vi "NumPad-ByRef.vi"(5 "Config":T1={"Title"="", "Minimum"=nan, "Maximum"=nan, "Decimals"=-1} {"Decimals" min=-1 max=6}, 6 "error in (no error)":errorcluster, 8 "device ID":refnum<k1>, 9 "NumericRef":refnum<vi>) -> (0 "error out":errorcluster, 2 "SetValue":dbl format="%#_8f", 3 "NumericRef out":refnum<vi>)   [LabVIEW 2016]
doc: "This subVI opens a number pad dialog to update the value to the referenced control.\nConfig cluster sets the title, max, min and number of decimal places. If config is not connected or any value is undefined, then the caption, max, min and increment of the referenced control are used.\n\nNOTE: The referenced control MUST have a caption set for LV8.5 !!!\n\n2-JAN-2008 R.Gibson"
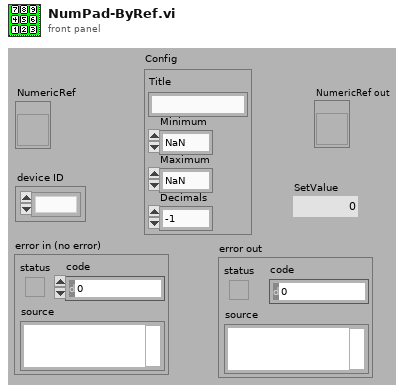
[diagram p1: front panel]
types:
  T1 = cluster{"Title":string, "Minimum":dbl, "Maximum":dbl, "Decimals":i8}
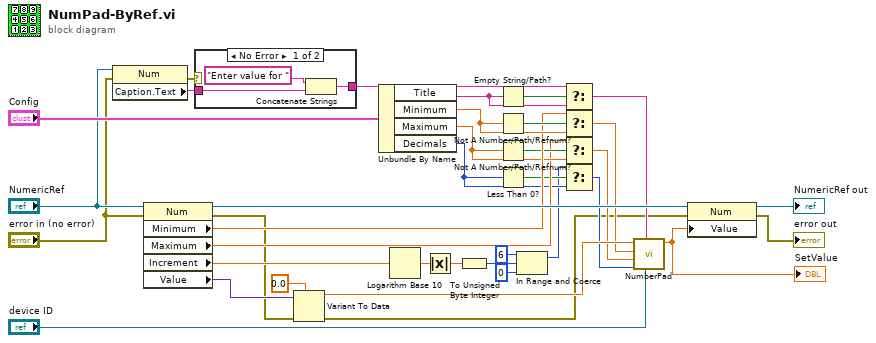
[diagram p0: block diagram]
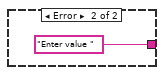
[diagram p2: hidden frame]
diagram:
  n1 = property on="Property Node" class="Num"(reference="NumericRef", error in="error in (no error)") -> (error out=w7:errorcluster, "Caption.Text"=w5:string)  [unwired: 1 out]
  n2 = property on="Property Node" class="Num"(reference="NumericRef", error in="error in (no error)") -> (reference out=w34:refnum<vi>, error out=w2:errorcluster, "Minimum"=w23:dbl, "Maximum"=w19:dbl, "Increment"=w35:dbl, "Value"=w6:variant)
  n3 = case shown="No Error" w7 {
    tunnel: w5 -> [w39 _]
    tunnel: [w38 "Enter value " ("Caption.Text")] -> w4
    frame No Error {
      n4 = Concatenate Strings("Enter value for " ("string"), w39) -> (w38:string)
    }
    frame Error {
    }
  }
  n5 = Variant To Data(error in=w2, type=0.0, Variant=w6) -> (data=w32:dbl, error out=w1:errorcluster)
  n6 = Unbundle By Name("Config") -> ("Title"=w27:string, "Minimum"=w24:dbl, "Maximum"=w20:dbl, "Decimals"=w16:i8)
  n7 = Logarithm Base 10(1:w35) -> (0:w36:dbl)
  n8 = Absolute Value(x=w36) -> (abs(x)=w14:dbl)
  n9 = To Unsigned Byte Integer(number=w14) -> (unsigned 8bit integer=w10:u8)
  n10 = Empty String/Path?(string/path=w27) -> (empty?=w28:bool)
  n11 = Not A Number/Path/Refnum?(number/path/refnum=w24) -> (NaN/Path/Refnum?=w25:bool)
  n12 = Not A Number/Path/Refnum?(number/path/refnum=w20) -> (NaN/Path/Refnum?=w21:bool)
  n13 = Less Than 0?(x=w16) -> (x < 0?=w15:bool)
  n14 = In Range and Coerce(upper limit=u8 6, x=w10, lower limit=u8 0) -> (coerced(x)=w13:u8)  [unwired: 1 out]
  n15 = Select(t=w4, s=w28, f=w27) -> (s? t:f=w26:string)
  n16 = Select(t=w23, s=w25, f=w24) -> (s? t:f=w22:dbl)
  n17 = Select(t=w19, s=w21, f=w20) -> (s? t:f=w18:dbl)
  n18 = Select(t=w13, s=w15, f=w16) -> (s? t:f=w17:u8)
  n19 = call "NumberPad.vi"("device ID"="device ID", "Window_Title"=w26, "Decimals (0)"=w17, "Max_Value (100)"=w18, "Min_Value (0)"=w22, "Default_Value (0)"=w32) -> ("Return_Value"=w31:dbl)  [unwired: 5 out]
  "SetValue" <- w31
  n20 = property on="Property Node" class="Num"(reference=w34, error in=w1, "Value"=w31) -> (reference out=→"NumericRef out":refnum<vi>, error out=→"error out":errorcluster)
